vi "_Get Target Object (Prot).vi"(8 "error in (no error)":errorcluster, 11 "IUnknown in":refnum<class "IUnknown.lvclass">) -> (0 "error out":errorcluster, 2 "Target Object":refnum<class "Interfaceable.lvclass">, 3 "IUnknown out":refnum<class "IUnknown.lvclass">)   [LabVIEW 2009, in "IUnknown.lvclass"]
doc: "Returns an object reference to the target object. Interface implementations should use this VI when implementing Interface methods. The \"target\" is the class an Interface implementation is designed for."
uses:
  IUnknown.lvclass
  Interfaceable Class/Interfaceable.lvclass
  IUnknown.lvclass/IUnknown.ctl
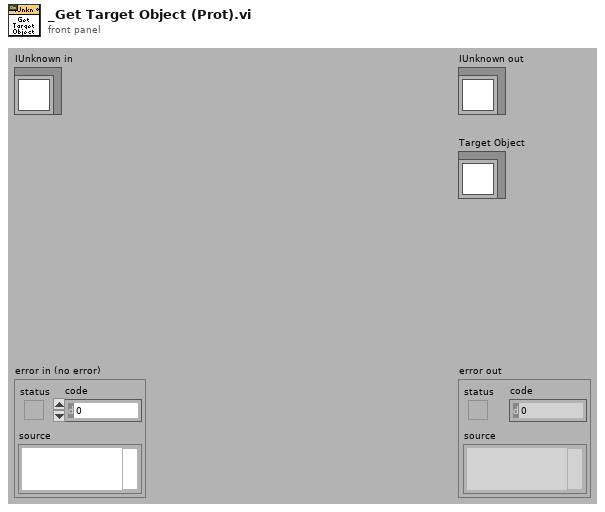
[diagram p1: front panel]
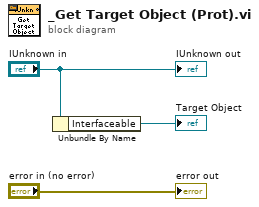
[diagram p0: block diagram]
diagram:
  n1 = Unbundle By Name("IUnknown in") -> ("Interfaceable"=→"Target Object":refnum<class "Interfaceable.lvclass">)
  "error out" <- "error in (no error)"
  "IUnknown out" <- "IUnknown in"
